vi "SynchronizationSaveTestWithTimer.vi"() -> ()   [LabVIEW 2019]
uses:
  C:/Users/Mastlab/Desktop/IMU VectorNAV VI/VectorNav.dll
  VectorNav.dll
panel:
  out "Magnetic.Z":dbl
  out "Magnetic.Y":dbl
  out "Magnetic.X":dbl
  in  "Path":path
  out "Timer":dbl
  out "Ready":bool
  out "Ending":bool
  out "Queue #":dbl
  in  "stop":bool
  out "Async Enable":bool
  out "Sensor Connected":bool
  out "Accel.Z":sgl
  out "Accel.Y":sgl
  out "Accel.X":sgl
  out "Gyro.Z":sgl
  out "Gyro.Y":sgl
  out "Gyro.X":sgl
  in  "Baudrate":string="115200"
  in  "COM Port":string="COM1"
  # "Note: Wait for 'Ready' to light up\nNote: Start Motion whitin 20 seconds after starting this VI"
  # "Data"
  # "Diagnostics"
  # "Output Table:\nAccel.X Accel.Y Accel.Z Gyro.X Gyro.Y Gyro.Z Magnetic.X Magnetic.Y Magnetic.Z  Quaternions\n               m/s^2                               rad/s                                             G                                      X Y Z W"
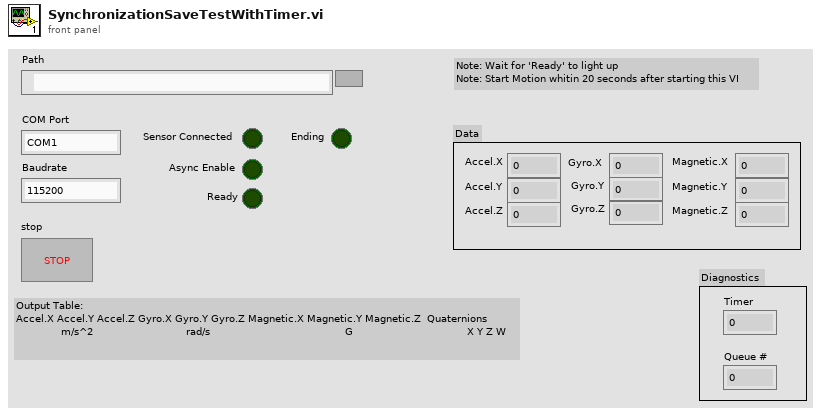
[diagram p1: front panel]
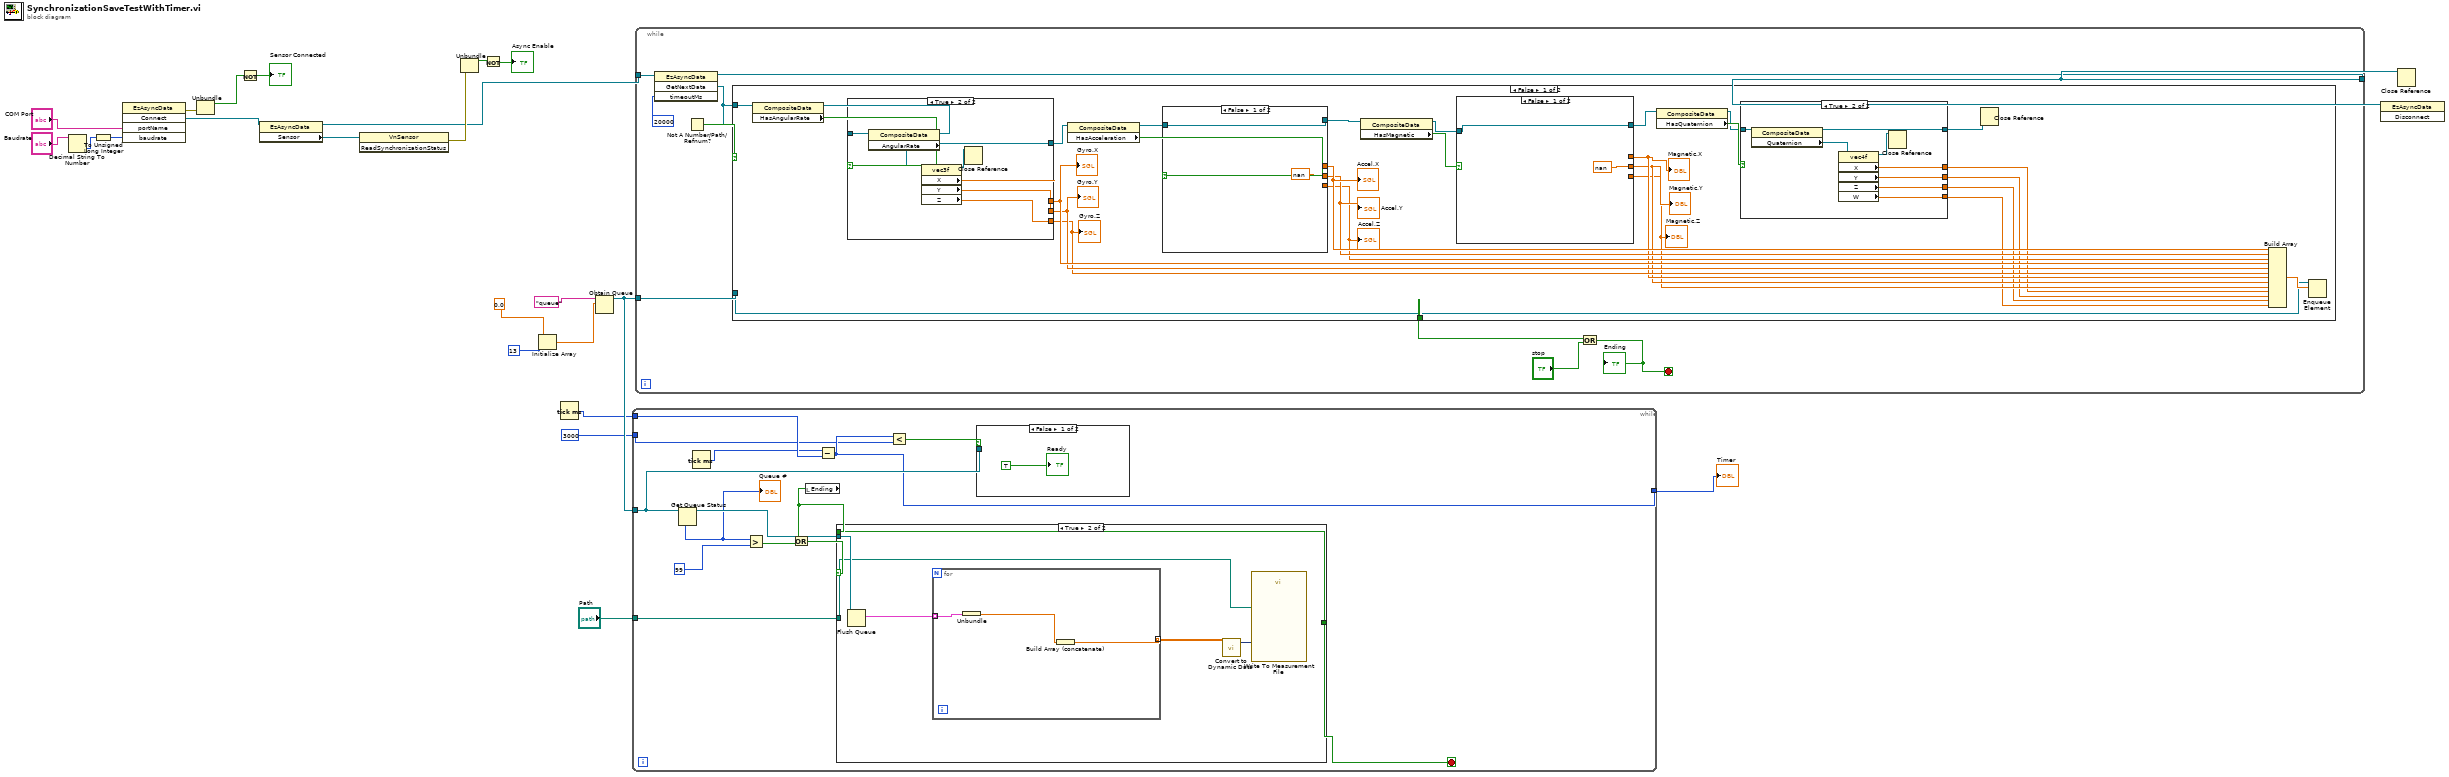
[diagram p0: block diagram]
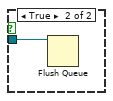
[diagram p2: hidden frame]
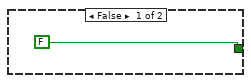
[diagram p3: hidden frame]
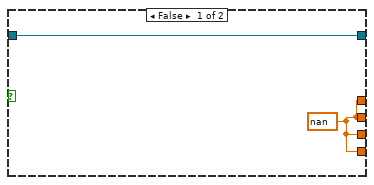
[diagram p4: hidden frame]
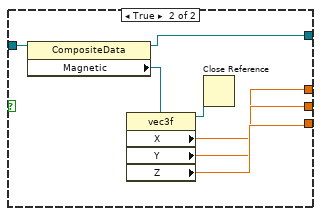
[diagram p5: hidden frame]
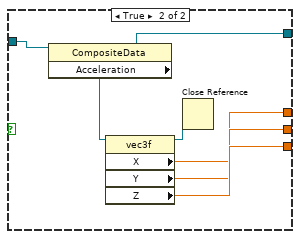
[diagram p6: hidden frame]
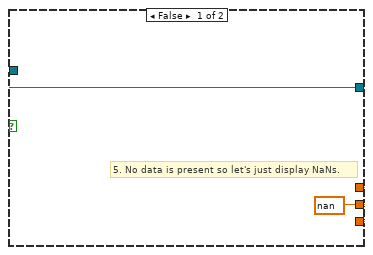
[diagram p7: hidden frame]
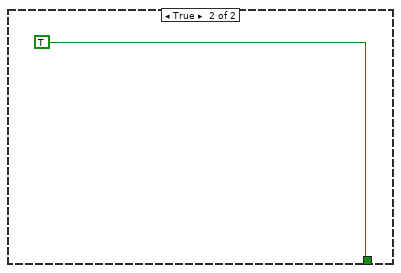
[diagram p8: hidden frame]
diagram:
  n1 = Decimal String To Number(string="Baudrate") -> (number=w23:i32)  [unwired: 2 in, 1 out]
  n2 = To Unsigned Long Integer(number=w23) -> (unsigned 32bit integer=w21:u32)
  n3 = invoke class="EzAsyncData" method="Connect"("portName"="COM Port", "baudrate"=w21) -> (error out=w19:errorcluster, "Connect"=w17:refnum<k24>)  [unwired: 3 in, 3 out]
  n4 = Unbundle(w19) -> ("status"=w18:bool)  [unwired: 2 out]
  n5 = Not(x=w18) -> (.not. x?=→"Sensor Connected":bool)
  n6 = property class="EzAsyncData"(reference=w17) -> (reference out=w6:refnum<k24>, "Sensor"=w16:refnum<k24>)  [unwired: 1 in, 1 out]
  n7 = invoke class="VnSensor" method="ReadSynchronizationStatus"(reference=w16) -> (error out=w15:errorcluster)  [unwired: 2 in, 2 out]
  n8 = Unbundle(w15) -> ("status"=w14:bool)  [unwired: 2 out]
  n9 = Not(x=w14) -> (.not. x?=→"Async Enable":bool)
  n10 = Initialize Array(0.0, 13) -> (w11:dbl[])
  n11 = Tick Count (ms)() -> (millisecond timer value=w4:u32)
  n12 = Obtain Queue(name (unnamed)="queue", element data type=w11) -> (queue out=w8:refnum<queue>)  [unwired: 3 in, 2 out]
  n13 = while {
    tunnel: w8 -> [w28]
    tunnel: 3000 -> [w25]
    tunnel: w4 -> [w30]
    tunnel: [w26] -> w3
    tunnel: "Path" -> [w27]
    stop <- w32 stop-if-true
    n14 = Get Queue Status(queue=w28) -> (queue out=w36:refnum<queue>, # elements in queue=w35:i32)  [unwired: 2 in, 6 out]
    "Queue #" <- w35
    n15 = Tick Count (ms)() -> (millisecond timer value=w29:u32)
    n16 = Greater?(x=w35, y=99) -> (0:w33:bool)
    n17 = local read "Ending"() -> (w31:bool)
    n18 = Or(x=w31, y=w33) -> (x .or. y?=w34:bool)
    n19 = Subtract(x=w29, y=w30) -> (x-y=w26:u32)
    n20 = case shown="True" w34 {
      tunnel: w36 -> [_ w46]
      tunnel: [FALSE w42] -> w32
      tunnel: w31 -> [_ w42]
      tunnel: w27 -> [_ w41]
      frame False {
      }
      frame True {
        n21 = Flush Queue(queue=w46) -> (remaining elements=w45:cluster{dbl[]}[])  [unwired: 1 in, 2 out]
        n22 = for {
          tunnel: w45 -> [w48] mode=indexing
          tunnel: [w49] -> w43 mode=indexing
          n23 = Unbundle(w48) -> (w47:dbl[])
          n24 = Build Array (concatenate)(w47) -> (w49:dbl[])
        }
        n25 = call "Convert to Dynamic Data"("2D Array"=w43) -> ("Dynamic Data Type"=w44:dynamicdata)  [unwired: 3 in]
        n26 = call "Write To Measurement File"("Signals"=w44, "Filename"=w41) -> ()  [unwired: 15 in, 3 out]
      }
    }
    n27 = Less?(x=w26, y=w25) -> (x < y?=w24:bool)
    n28 = case shown="False" w24 {
      tunnel: w28 -> [_ w39]
      frame False {
        "Ready" <- TRUE
      }
      frame True {
        n29 = Flush Queue(queue=w39) -> ()  [unwired: 1 in, 3 out]
      }
    }
  }
  "Timer" <- w3
  n30 = while {
    tunnel: [w58] -> w13
    tunnel: w8 -> [w56]
    tunnel: w6 -> [w53]
    stop <- w54 stop-if-true
    n31 = invoke class="EzAsyncData" method="GetNextData"(reference=w53, "timeoutMs"=20000) -> (reference out=w58:refnum<k24>, "GetNextData"=w50:refnum<k24>)  [unwired: 2 in, 2 out]
    n32 = Not A Number/Path/Refnum?(number/path/refnum=w50) -> (NaN/Path/Refnum?=w51:bool)
    n33 = case shown="False" w51 {
      tunnel: w50 -> [w82 _]
      tunnel: [_ TRUE] -> w55
      tunnel: w56 -> [w78 _]
      frame False {
        n34 = property on="Property Node" class="CompositeData"(reference=w82) -> (reference out=w85:refnum<k24>, "HasAngularRate"=w86:bool)  [unwired: 1 in, 1 out]
        n35 = case shown="True" w86 {
          tunnel: w85 -> [w115 w118]
          tunnel: [w116 w119] -> w76
          tunnel: [w116 w120] -> w75
          tunnel: [w116 w121] -> w74
          tunnel: [w115 w123] -> w84
          frame False {
            w116 = sgl nan
            # "5. No data is present so let's just display NaNs."
          }
          frame True {
            n36 = property class="CompositeData"(reference=w118) -> (reference out=w123:refnum<k24>, "AngularRate"=w117:refnum<k24>)  [unwired: 1 in, 1 out]
            n37 = property class="vec3f"(reference=w117) -> (reference out=w122:refnum<k24>, "X"=w119:sgl, "Y"=w120:sgl, "Z"=w121:sgl)  [unwired: 1 in, 1 out]
            n38 = Close Reference(reference=w122) -> ()  [unwired: 1 in, 1 out]
          }
        }
        "Gyro.X" <- w76
        "Gyro.Y" <- w75
        "Gyro.Z" <- w74
        n39 = property class="CompositeData"(reference=w84) -> (reference out=w65:refnum<k24>, "HasAcceleration"=w83:bool)  [unwired: 1 in, 1 out]
        n40 = case shown="False" w83 {
          tunnel: [w107 w110] -> w81
          tunnel: [w107 w111] -> w80
          tunnel: [w107 w112] -> w77
          tunnel: [w106 w114] -> w64
          tunnel: w65 -> [w106 w108]
          frame False {
            w107 = sgl nan
          }
          frame True {
            n41 = property class="CompositeData"(reference=w108) -> (reference out=w114:refnum<k24>, "Acceleration"=w113:refnum<k24>)  [unwired: 1 in, 1 out]
            n42 = property class="vec3f"(reference=w113) -> (reference out=w109:refnum<k24>, "X"=w110:sgl, "Y"=w111:sgl, "Z"=w112:sgl)  [unwired: 1 in, 1 out]
            n43 = Close Reference(reference=w109) -> ()  [unwired: 1 in, 1 out]
          }
        }
        "Accel.X" <- w81
        "Accel.Y" <- w80
        "Accel.Z" <- w77
        n44 = property class="CompositeData"(reference=w64) -> (reference out=w73:refnum<k24>, "HasMagnetic"=w66:bool)  [unwired: 1 in, 1 out]
        n45 = case shown="False" w66 {
          tunnel: [w98 w101] -> w72
          tunnel: [w98 w102] -> w71
          tunnel: [w98 w103] -> w70
          tunnel: [w97 w105] -> w69
          tunnel: w73 -> [w97 w99]
          frame False {
            w98 = sgl nan
          }
          frame True {
            n46 = property class="CompositeData"(reference=w99) -> (reference out=w105:refnum<k24>, "Magnetic"=w104:refnum<k24>)  [unwired: 1 in, 1 out]
            n47 = property class="vec3f"(reference=w104) -> (reference out=w100:refnum<k24>, "X"=w101:sgl, "Y"=w102:sgl, "Z"=w103:sgl)  [unwired: 1 in, 1 out]
            n48 = Close Reference(reference=w100) -> ()  [unwired: 1 in, 1 out]
          }
        }
        "Magnetic.X" <- w72
        "Magnetic.Y" <- w71
        "Magnetic.Z" <- w70
        n49 = property class="CompositeData"(reference=w69) -> (reference out=w67:refnum<k24>, "HasQuaternion"=w68:bool)  [unwired: 1 in, 1 out]
        n50 = case shown="True" w68 {
          tunnel: w67 -> [w87 w96]
          tunnel: [w88 w93] -> w63
          tunnel: [w88 w92] -> w62
          tunnel: [w88 w91] -> w61
          tunnel: [w88 w90] -> w60
          tunnel: [w87 w89] -> w59
          frame False {
            w88 = sgl nan
          }
          frame True {
            n51 = property class="CompositeData"(reference=w96) -> (reference out=w89:refnum<k24>, "Quaternion"=w95:refnum<k24>)  [unwired: 1 in, 1 out]
            n52 = property class="vec4f"(reference=w95) -> (reference out=w94:refnum<k24>, "X"=w93:sgl, "Y"=w92:sgl, "Z"=w91:sgl, "W"=w90:sgl)  [unwired: 1 in, 1 out]
            n53 = Close Reference(reference=w94) -> ()  [unwired: 1 in, 1 out]
          }
        }
        n54 = Close Reference(reference=w59) -> ()  [unwired: 1 in, 1 out]
        n55 = Build Array(w81, w80, w77, w76, w75, w74, w72, w71, w70, w63, w62, w61, w60) -> (w79:sgl[])
        n56 = Enqueue Element(queue=w78, element=w79) -> ()  [unwired: 2 in, 3 out]
      }
      frame True {
      }
    }
    n57 = Or(x=w55, y="stop") -> (x .or. y?=w54:bool)
    "Ending" <- w54
  }
  n58 = invoke class="EzAsyncData" method="Disconnect"(reference=w13) -> ()  [unwired: 2 in, 3 out]
  n59 = Close Reference(reference=w13) -> ()  [unwired: 1 in, 1 out]
